vi "Caesar-Cipher.vi"() -> ()   [LabVIEW 2014]
panel:
  in  "Switch":bool
  in  "Shift":i32
  out "Output string":string
  in  "Input string":string
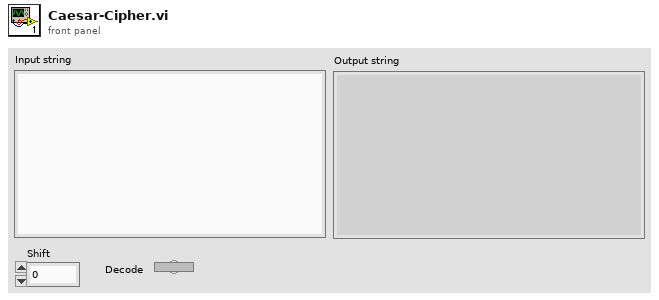
[diagram p1: front panel]
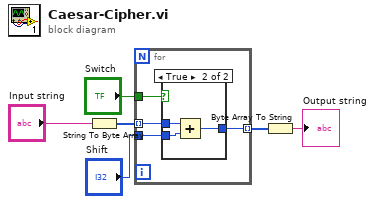
[diagram p0: block diagram]
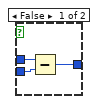
[diagram p2: hidden frame]
diagram:
  n1 = String To Byte Array(string="Input string") -> (unsigned byte array=w3:u8[])
  n2 = for {
    tunnel: "Switch" -> [w10]
    tunnel: "Shift" -> [w9]
    tunnel: w3 -> [w8] mode=indexing
    tunnel: [w7] -> w2 mode=indexing
    n3 = case shown="True" w10 {
      tunnel: w9 -> [w11 w16]
      tunnel: w8 -> [w12 w15]
      tunnel: [w13 w14] -> w7
      frame False {
        n4 = Subtract(x=w12, y=w11) -> (x-y=w13:i32)
      }
      frame True {
        n5 = Add(x=w15, y=w16) -> (x+y=w14:i32)
      }
    }
  }
  n6 = Byte Array To String(unsigned byte array=w2) -> (string=→"Output string":string)
